vi "Configure Module.vi"(8 "error in (no error)":errorcluster, 10 "IOV ref in":refnum<k21>, 11 "RSI Module in":refnum<class "RSI Module.lvclass">) -> (0 "error out":errorcluster, 2 "IOV ref out":refnum<k21>, 3 "RSI Module out":refnum<class "RSI Module.lvclass">)   [LabVIEW 2017, in "Modules.lvlib" / "RSI Module.lvclass"]
uses:
  RSI Module.lvclass
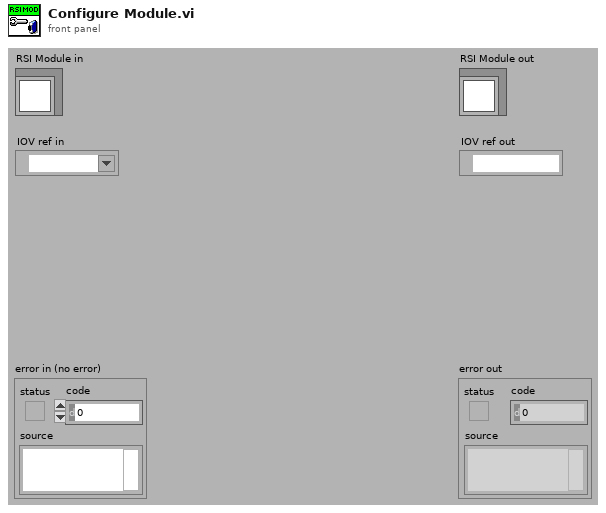
[diagram p1: front panel]
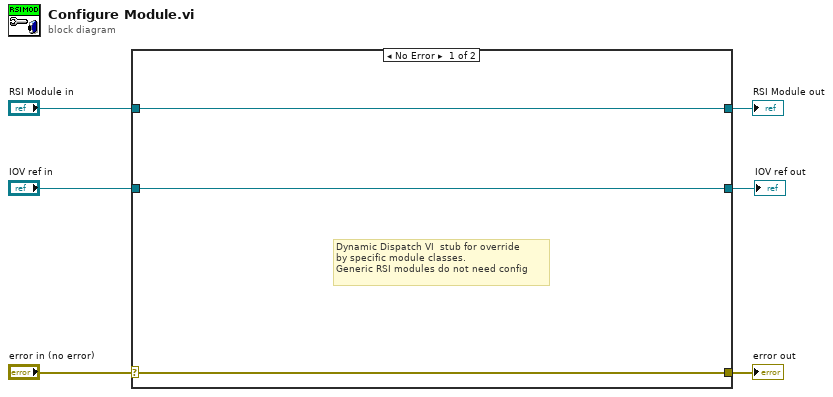
[diagram p0: block diagram]
diagram:
  n1 = case shown="No Error" "error in (no error)" {
    selector: "error in (no error)" -> [w8 w12]
    tunnel: [w8 w12] -> w5
    tunnel: [w9 w11] -> w3
    tunnel: "RSI Module in" -> [w9 w11]
    tunnel: "IOV ref in" -> [w7 w10]
    tunnel: [w7 w10] -> w1
    frame No Error {
      # "Dynamic Dispatch VI  stub for override\nby specific module classes.\nGeneric RSI modules do not need config"
    }
    frame Error {
    }
  }
  "error out" <- w5
  "RSI Module out" <- w3
  "IOV ref out" <- w1
